vi "Felix Event FSM Template.vi"() -> ()   [LabVIEW 2017]
panel:
  in  "Loop Back":bool
  in  "Skip Step 2":bool
  out "FSM State":string
  out "LED 2.3":bool
  out "LED 2.2":bool
  out "LED 2.1":bool
  out "LED 1.3":bool
  out "LED 1.2":bool
  out "LED 1.1":bool
  in  "Start Sequence 2":bool
  in  "Start Sequence 1":bool
  in  "stop":bool
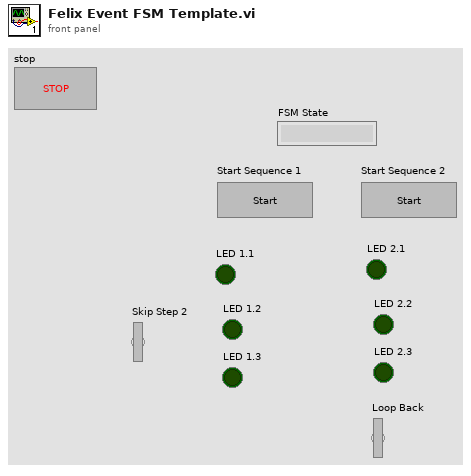
[diagram p1: front panel]
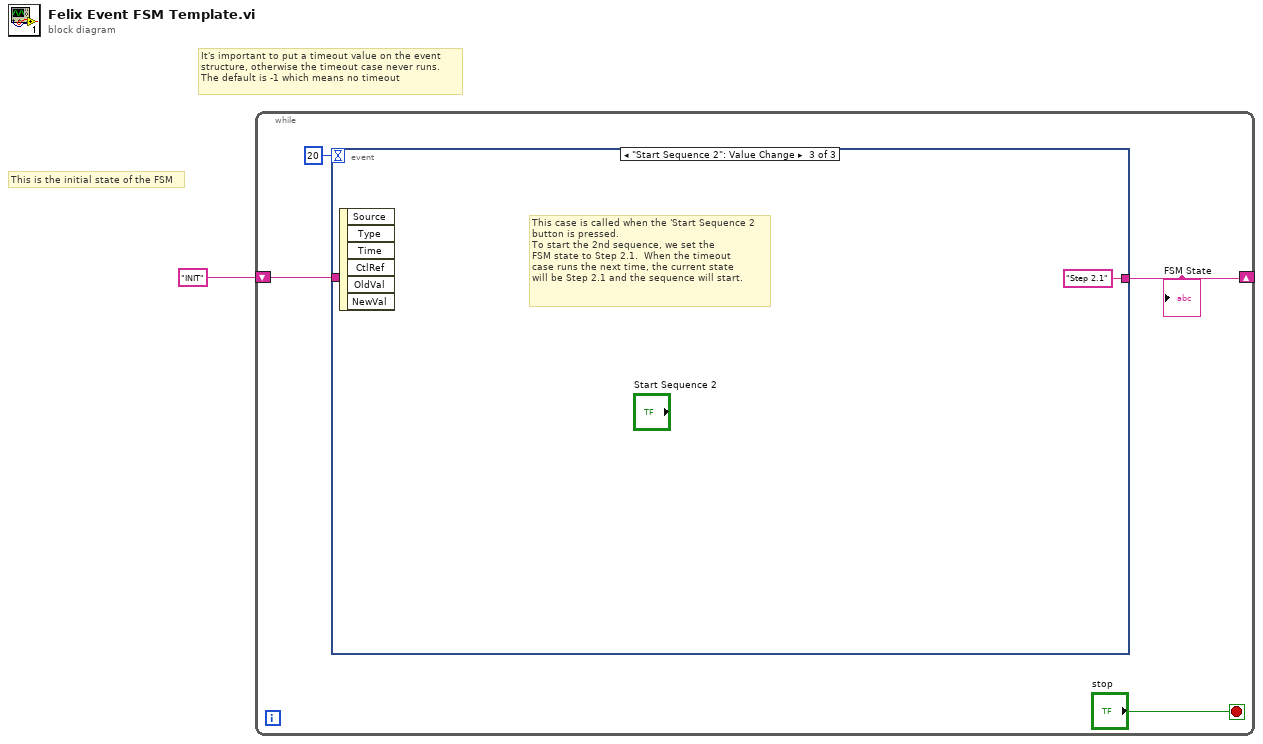
[diagram p0: block diagram]
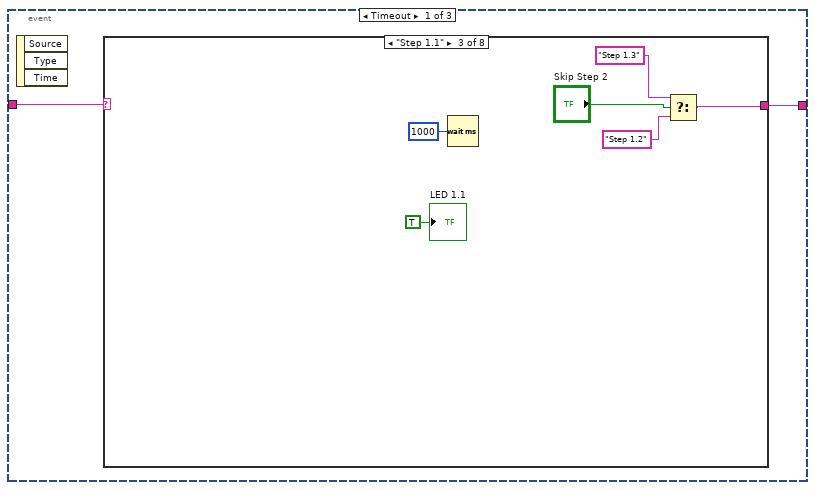
[diagram p2: hidden frame]
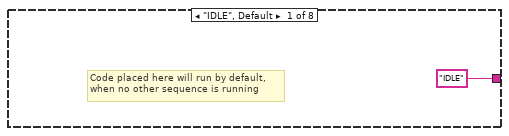
[diagram p3: hidden frame]
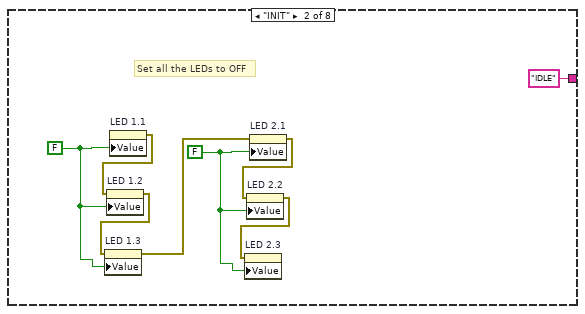
[diagram p4: hidden frame]
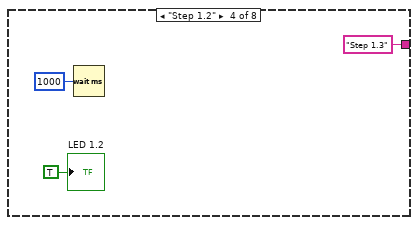
[diagram p5: hidden frame]
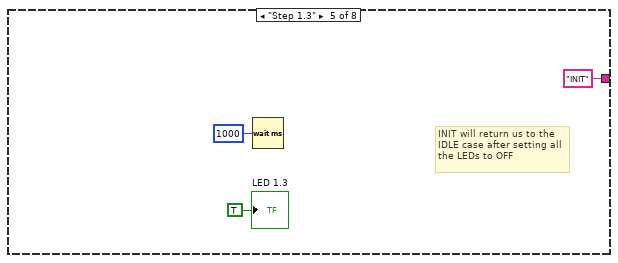
[diagram p6: hidden frame]
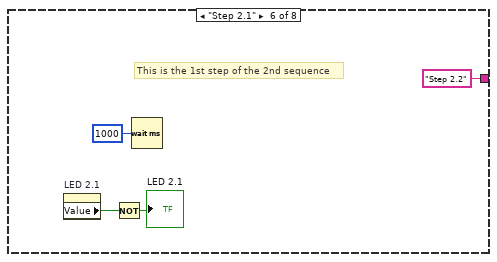
[diagram p7: hidden frame]
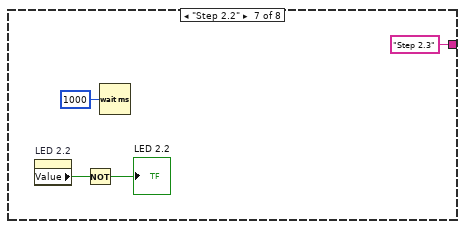
[diagram p8: hidden frame]
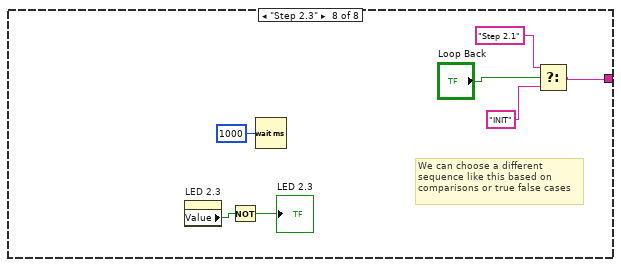
[diagram p9: hidden frame]
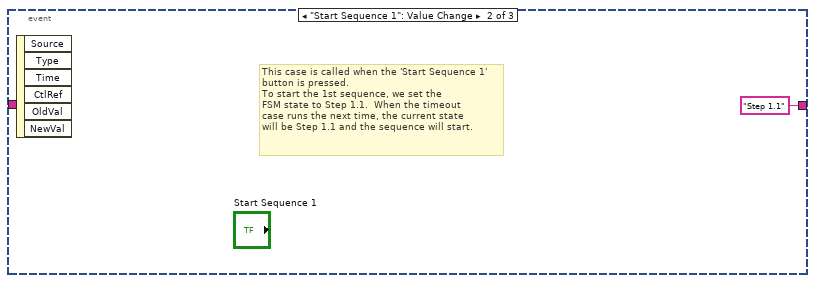
[diagram p10: hidden frame]
diagram:
  # "This is the initial state of the FSM"
  # "It's important to put a timeout value on the event\nstructure, otherwise the timeout case never runs. \nThe default is -1 which means no timeout"
  n1 = while {
    shift-right: [w4] -> _
    shift-left: "INIT" -> [w5]
    stop <- "stop" stop-if-true
    n2 = event shown="[2] \"Start Sequence 2\": Value Change" {
      selector: _ -> [_ _ _]
      dyn-events: _ -> [_ _ _]
      timeout: 20 -> [_ _ _]
      tunnel: w5 -> [w7 _ _]
      tunnel: [w6 "Step 1.1" ("f") "Step 2.1" ("f")] -> w4
      event Timeout {
        n3 = event-data() -> ()  [unwired: 1 in, 3 out]
        n4 = case shown="\"Step 1.1\"" w7 {
          tunnel: ["IDLE" "IDLE" w19 "Step 1.3" "INIT" "Step 2.2" "Step 2.3" w41] -> w6
          frame "IDLE", Default {
            # "Code placed here will run by default,\nwhen no other sequence is running"
          }
          frame "INIT" {
            w10 = FALSE ("LED 2.1")
            w15 = FALSE ("LED 2.1")
            # "Set all the LEDs to OFF"
            n5 = property on="LED 1.1" class="Bool (strict)"("Value"=w15) -> (error out=w14:errorcluster)  [unwired: 2 in, 1 out]
            n6 = property on="LED 1.2" class="Bool (strict)"(error in=w14, "Value"=w15) -> (error out=w13:errorcluster)  [unwired: 1 in, 1 out]
            n7 = property on="LED 1.3" class="Bool (strict)"(error in=w13, "Value"=w15) -> (error out=w9:errorcluster)  [unwired: 1 in, 1 out]
            n8 = property on="LED 2.1" class="Bool (strict)"(error in=w9, "Value"=w10) -> (error out=w11:errorcluster)  [unwired: 1 in, 1 out]
            n9 = property on="LED 2.2" class="Bool (strict)"(error in=w11, "Value"=w10) -> (error out=w12:errorcluster)  [unwired: 1 in, 1 out]
            n10 = property on="LED 2.3" class="Bool (strict)"(error in=w12, "Value"=w10) -> ()  [unwired: 1 in, 2 out]
          }
          frame "Step 1.1" {
            n11 = Wait (ms)(milliseconds to wait=u32 1000) -> ()  [unwired: 1 out]
            n12 = Select(t="Step 1.3", s="Skip Step 2", f="Step 1.2") -> (s? t:f=w19:string)
            "LED 1.1" <- TRUE ("LED 1.1")
          }
          frame "Step 1.2" {
            n13 = Wait (ms)(milliseconds to wait=u32 1000) -> ()  [unwired: 1 out]
            "LED 1.2" <- TRUE ("LED 1.2")
          }
          frame "Step 1.3" {
            # "INIT will return us to the\nIDLE case after setting all\nthe LEDs to OFF"
            n14 = Wait (ms)(milliseconds to wait=u32 1000) -> ()  [unwired: 1 out]
            "LED 1.3" <- TRUE ("LED 1.3")
          }
          frame "Step 2.1" {
            # "This is the 1st step of the 2nd sequence"
            n15 = property on="LED 2.1" class="Bool (strict)"() -> ("Value"=w30:bool)  [unwired: 2 in, 2 out]
            n16 = Not(x=w30) -> (.not. x?=→"LED 2.1":bool)
            n17 = Wait (ms)(milliseconds to wait=u32 1000) -> ()  [unwired: 1 out]
          }
          frame "Step 2.2" {
            n18 = property on="LED 2.2" class="Bool (strict)"() -> ("Value"=w34:bool)  [unwired: 2 in, 2 out]
            n19 = Not(x=w34) -> (.not. x?=→"LED 2.2":bool)
            n20 = Wait (ms)(milliseconds to wait=u32 1000) -> ()  [unwired: 1 out]
          }
          frame "Step 2.3" {
            # "We can choose a different\nsequence like this based on\ncomparisons or true false cases"
            n21 = property on="LED 2.3" class="Bool (strict)"() -> ("Value"=w38:bool)  [unwired: 2 in, 2 out]
            n22 = Not(x=w38) -> (.not. x?=→"LED 2.3":bool)
            n23 = Wait (ms)(milliseconds to wait=u32 1000) -> ()  [unwired: 1 out]
            n24 = Select(t="Step 2.1", s="Loop Back", f="INIT") -> (s? t:f=w41:string)
          }
        }
      }
      event "Start Sequence 1": Value Change {
        # "This case is called when the 'Start Sequence 1'\nbutton is pressed.\nTo start the 1st sequence, we set the \nFSM state to Step 1.1.  When the timeout\ncase runs the next time, the current state\nwill be Step 1.1 and the sequence will start."
        n25 = event-data() -> ()  [unwired: 1 in, 6 out]
      }
      event "Start Sequence 2": Value Change {
        # "This case is called when the 'Start Sequence 2\nbutton is pressed.\nTo start the 2nd sequence, we set the \nFSM state to Step 2.1.  When the timeout\ncase runs the next time, the current state\nwill be Step 2.1 and the sequence will start."
        n26 = event-data() -> ()  [unwired: 1 in, 6 out]
      }
    }
    "FSM State" <- w4
  }
